vi "5_1.vi"() -> ()   [LabVIEW 2020]
panel:
  out "Drehspulinstrument":dbl(knob) caption="Spule" scale=0.0..10.0
  in  "Schieberegler":dbl(slide) caption="Regler" scale=0.0..10.0
  out "Boolesch":bool caption="LED"
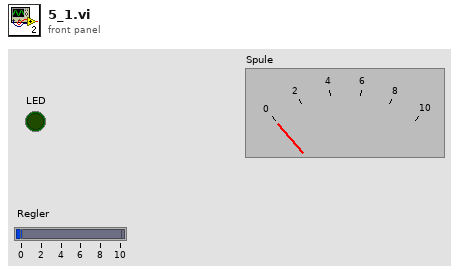
[diagram p1: front panel]
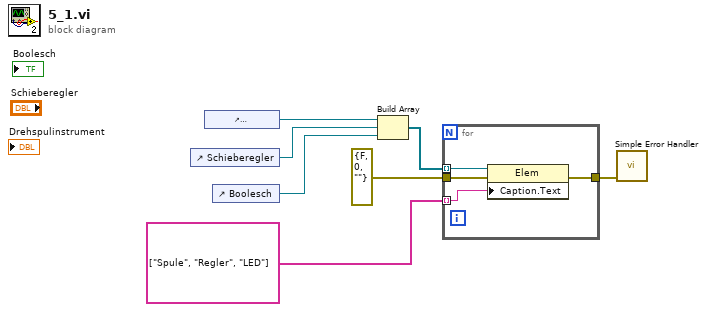
[diagram p0: block diagram]
diagram:
  n1 = control-ref of="Schieberegler"() -> (w6:refnum<vi>)
  n2 = control-ref of="Drehspulinstrument"() -> (w7:refnum<vi>)
  n3 = control-ref of="Boolesch"() -> (w5:refnum<vi>)
  n4 = Build Array(w7, w6, w5) -> (w4:refnum<vi>[])
  n5 = for {
    tunnel: w4 -> [w11] mode=indexing
    tunnel: string[] ["Spule", "Regler", "LED"] -> [w10] mode=indexing
    tunnel: errorcluster {"status"=FALSE, "code"=0, "source"=""} ("Fehler (Eingang, kein Fehler)") -> [w9]
    tunnel: [w8] -> w1
    n6 = property class="Elem"(reference=w11, error in=w9, "Caption.Text"=w10) -> (error out=w8:errorcluster)  [unwired: 1 out]
  }
  n7 = call <vilib>:"Simple Error Handler.vi"("error in (no error)"=w1) -> ()  [unwired: 4 in, 5 out]
